vi "Handle Error.vi"(8 "error in (no error)":errorcluster, 11 "AdvancedActor in":refnum<class "AdvancedActor.lvclass">) -> (0 "error out":errorcluster, 2 "stop actor?":bool=TRUE, 3 "AdvancedActor out":refnum<class "AdvancedActor.lvclass">)   [LabVIEW 2020, in "MGI-Panel Actor.lvlib" / "AdvancedActor.lvlib" / "AdvancedActor.lvclass"]
doc: "(<B>Filename</B>: Actor Framework.lvlib:Actor.lvclass:Handle Error.vi)\n\nDefines how the actor handles an error that occurred while processing a message. By default, this method does nothing except stop the actor."
uses:
  AdvancedActor.lvclass
  C:/Program Files (x86)/National Instruments/LabVIEW 2020/vi.lib/ActorFramework/Actor/Actor.lvclass
  AdvancedActor Messages/ShutdownTimedOut Msg/ShutdownTimedOut Msg.lvclass
  C:/Program Files (x86)/National Instruments/LabVIEW 2020/vi.lib/ActorFramework/Message/Message.lvclass
  <vilib>/ActorFramework/Actor/Actor.lvclass/Actor.ctl
  <vilib>/ActorFramework/Message Enqueuer/Message Enqueuer.lvclass/Message Enqueuer.ctl
  AdvancedActor.lvclass/AdvancedActor.ctl
  <vilib>/ActorFramework/Time-Delayed Send Message/Time-Delay Override Options.ctl
  <vilib>/ActorFramework/Message Enqueuer/Init from Existing Queue.vi
  <vilib>/ActorFramework/Message Enqueuer/Message Enqueuer.lvclass
  <vilib>/ErrorRing/Error Ring.xnode
  <vilib>/Utility/error.llb/Error Cluster From Error Code.vi
  <vilib>/ActorFramework/Actor/Actor.lvclass
  D:/test/LabView_PanelManager/panel-actors/Source/AdvancedActor/AdvancedActor Messages/ShutdownTimedOut Msg/ShutdownTimedOut Msg.lvclass
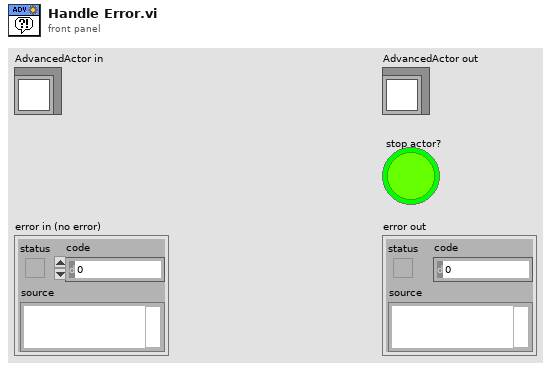
[diagram p1: front panel]
types:
  T1 = typedef "Time-Delay Override Options.ctl" = enum16{"Send next copy now", "Skip next scheduled copy", "Send next copy now and stop all further copies", "Stop all further copies"}
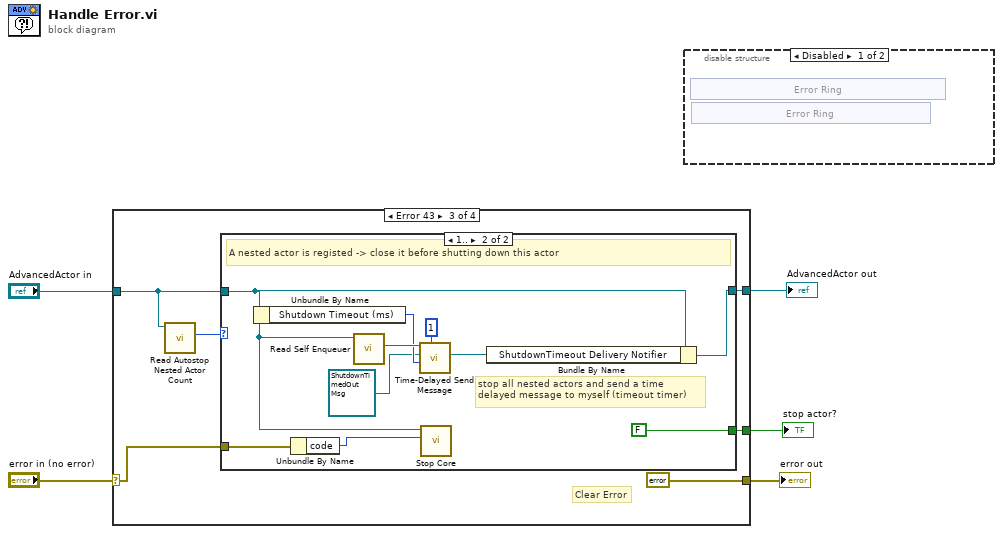
[diagram p0: block diagram]
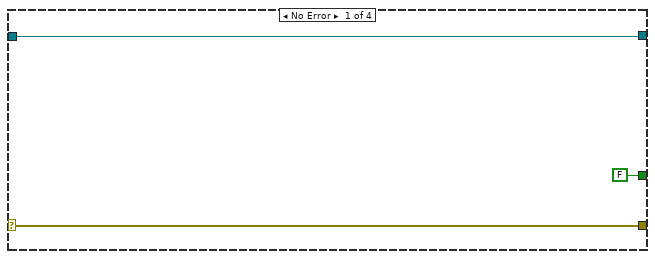
[diagram p3: hidden frame]
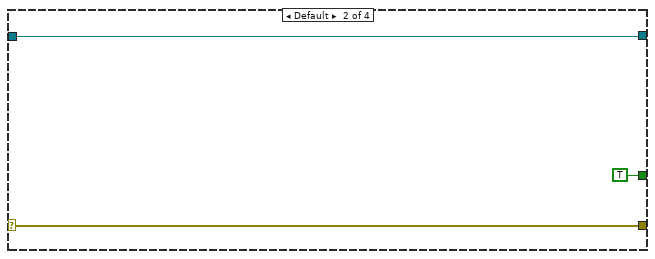
[diagram p4: hidden frame]
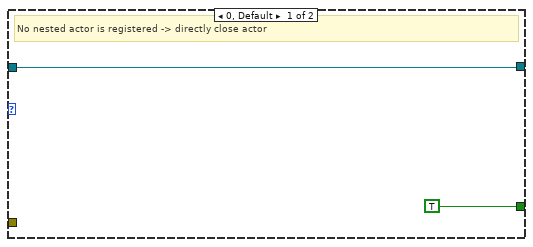
[diagram p5: hidden frame]
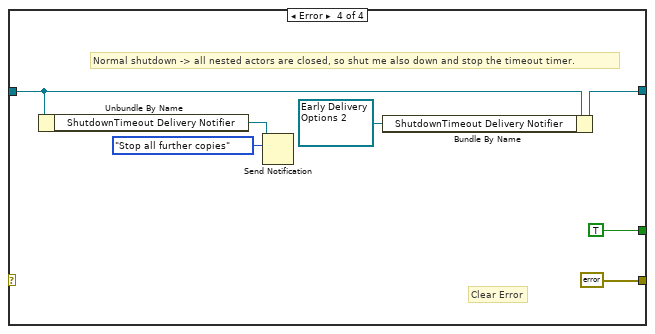
[diagram p6: hidden frame]
diagram:
  n1 = case shown="Error 43" "error in (no error)" {
    selector: "error in (no error)" -> [w8 w11 w12 _]
    tunnel: [w8 w11 errorcluster {"status"=FALSE, "code"=0, "source"=""} ("error IO") errorcluster {"status"=FALSE, "code"=0, "source"=""} ("error IO")] -> w4
    tunnel: [FALSE TRUE w14 TRUE] -> w3
    tunnel: "AdvancedActor in" -> [w6 w9 w15 w32]
    tunnel: [w6 w9 w13 w34] -> w1
    frame No Error {
    }
    frame Default {
    }
    frame Error {
      # "Clear Error"
      n2 = call <vilib>:"Read Autostop Nested Actor Count.vi"("Actor in"=w15) -> ("Count"=w16:i32)  [unwired: 10 in]
      n3 = case shown="1.." w16 {
        tunnel: w15 -> [w18 w24]
        tunnel: [TRUE FALSE] -> w14
        tunnel: [w18 w23] -> w13
        tunnel: w12 -> [_ w21]
        frame 0, Default {
          # "No nested actor is registered -> directly close actor"
        }
        frame 1.. {
          # "stop all nested actors and send a time\ndelayed message to myself (timeout timer)"
          # "A nested actor is registed -> close it before shutting down this actor"
          n4 = Unbundle By Name(w24) -> ("Shutdown Timeout (ms)"=w27:i32)
          n5 = Unbundle By Name(w21) -> ("code"=w20:i32)
          n6 = call <vilib>:"Read Self Enqueuer.vi"("Actor"=w24) -> ("Self Enqueuer"=w29:refnum<class "Message Enqueuer.lvclass">)  [unwired: 10 in]
          n7 = call <vilib>:"Time-Delayed Send Message.vi"("# Copies (0 = infinite repeat)"=u32 1, "Milliseconds To Wait"=w27, "Message"=refnum<class "ShutdownTimedOut Msg.lvclass"> refnum ("AdvancedActor.lvlib:ShutdownTimedOut Msg.lvclass"), "Message Enqueuer"=w29) -> ("Delivery Notifier"=w25:refnum<notifier>)  [unwired: 6 in, 1 out]
          n8 = call-dynamic "Stop Core.vi"("final error code"=w20, "Actor in"=w24) -> ()  [unwired: 9 in, 1 out]
          n9 = Bundle By Name(cluster=w24, "ShutdownTimeout Delivery Notifier"=w25) -> (w23:refnum<class "AdvancedActor.lvclass">)
        }
      }
    }
    frame Error {
      w33 = refnum<notifier> refnum items=["Send next copy now", "Skip next scheduled copy", "Send next copy now and stop all further copies", "Stop all further copies"] ("ShutdownTimeout Delivery Notifier")
      # "Normal shutdown -> all nested actors are closed, so shut me also down and stop the timeout timer."
      # "Clear Error"
      n10 = Unbundle By Name(w32) -> ("ShutdownTimeout Delivery Notifier"=w31:refnum<notifier>)
      n11 = Send Notification(notification=Time-Delay_Override_Options."Stop all further copies", notifier=w31) -> ()  [unwired: 1 in, 2 out]
      n12 = Bundle By Name(cluster=w32, "ShutdownTimeout Delivery Notifier"=w33) -> (w34:refnum<class "AdvancedActor.lvclass">)
    }
  }
  "AdvancedActor out" <- w1
  "error out" <- w4
  "stop actor?" <- w3
  n13 = disable-structure shown="Disabled" {
    frame Disabled {
      n14 = xnode "Error Ring"() -> ()  [unwired: 1 out]
      n15 = xnode "Error Ring"() -> ()  [unwired: 1 out]
    }
    frame Enabled {
    }
  }
